vi "Audio.Discover Devices by Name.vi"(8 "Error if Out Dev Not Found":bool, 9 "Output Device":string, 10 "Error if In Dev Not Found":bool, 11 "Input Device":string) -> (0 "Out Dev Found":bool, 1 "Out ID":i32, 2 "In Dev Found":bool, 3 "In ID":i32, 4 "error out":errorcluster)   [LabVIEW 2018]
uses:
  Utils/Errors/Error.Error Code List.ctl
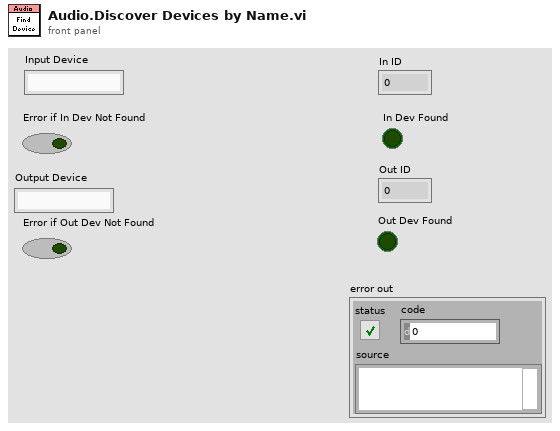
[diagram p1: front panel]
types:
  T1 = typedef "Error.Error Code List.ctl" = i32
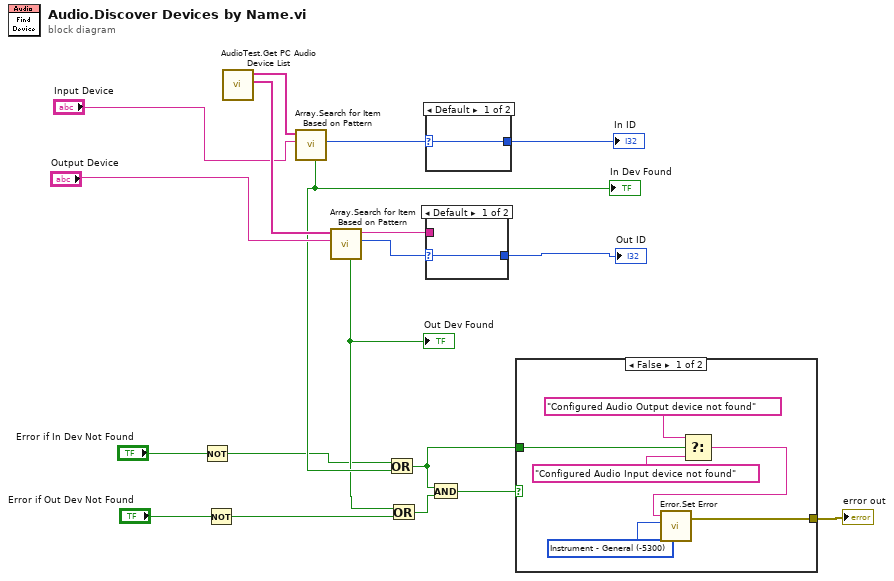
[diagram p0: block diagram]
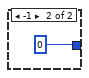
[diagram p3: hidden frame]
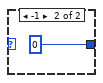
[diagram p4: hidden frame]
diagram:
  n1 = Not(x="Error if In Dev Not Found") -> (.not. x?=w4:bool)
  n2 = Not(x="Error if Out Dev Not Found") -> (.not. x?=w6:bool)
  n3 = call "AudioTest.Get PC Audio Device List.vi"() -> ("Output Devices"=w16:string[], "Input Devices"=w15:string[])  [unwired: 10 in]
  n4 = call "Array.Search for Item Based on Pattern.vi"("Pattern"="Input Device", "List"=w15) -> ("Index"=w17:i32, "Found"=w9:bool)  [unwired: 7 in, 1 out]
  "In Dev Found" <- w9
  n5 = call "Array.Search for Item Based on Pattern.vi"("Pattern"="Output Device", "List"=w16) -> ("Index"=w19:i32, "Found Item"=w18:string, "Found"=w8:bool)  [unwired: 7 in]
  "Out Dev Found" <- w8
  n6 = Or(x=w4, y=w9) -> (x .or. y?=w1:bool)
  n7 = Or(x=w8, y=w6) -> (x .or. y?=w3:bool)
  n8 = case shown="Default" w17 {
    selector: w17 -> [w20 _]
    tunnel: [w20 0 ("lower limit")] -> w11
    frame Default {
    }
    frame -1 {
    }
  }
  "In ID" <- w11
  n9 = case shown="Default" w19 {
    selector: w19 -> [w22 _]
    tunnel: [w22 0] -> w10
    tunnel: w18 -> [_ _]
    frame Default {
    }
    frame -1 {
    }
  }
  "Out ID" <- w10
  n10 = And(x=w1, y=w3) -> (x .and. y?=w14:bool)
  n11 = case shown="False" w14 {
    tunnel: w1 -> [w28 _]
    tunnel: [w24 _] -> w2
    frame False {
      w25 = T1 -5300 items=["No Error"=0, "Abort"=-2, "Misc"=-5000, "Fixture Error"=-5100, "File IO - General"=-5200, "FIle IO - Config Error"=-5201, "Instrument - General"=-5300, "Instrument - Serial Com"=-5301, "Instrument - Camera"=-5302, "Instrument - PS"=-5303, "Instrument - Oscilloscope"=-5304, "Instrument - Function Gen"=-5305, "Instrument - Load"=-5306, "Instrument - Meter"=-5307, "Instrument - Power Control"=-5308, "Instrument - Motion"=-5309, "Instrument - RF"=-5310, "System Exe"=-5400, "Image Processing"=-5500, "Communication"=-5600, "Script - Syntax Error"=-6000, "Script - Invalid Name or Param"=-6100, "Script - Timeout"=-6200, "Invalid Data"=-6300, "FW Update Error"=-6500] ("Std Code")
      n12 = Select(t="Configured Audio Output device not found", s=w28, f="Configured Audio Input device not found") -> (s? t:f=w26:string)
      n13 = call "Error.Set Error.vi"("Code"=w25, "Desc"=w26) -> ("error out"=w24:errorcluster)  [unwired: 5 in]
    }
    frame True {
    }
  }
  "error out" <- w2
